vi "MCA_ConfigDialog.vi"(0 "测量最多花费的时间（秒）：":u16=3600, 1 "测量数据刷新频率（个/次）：":u32, 2 "数据文件路径":path, 3 "道数":enum32{"1024", "2048", "4096", "8192"}(radio), 4 "输入信号的极性：":enum32{"正", "负"}(radio), 5 "寻峰灵敏度：":u16=30 min=3 step=1, 6 "甄别前阈值":u16=200, 7 "甄别后阈值":u16=100) -> (14 "输入信号极性":bool, 16 "甄别后阈值 2":dbl=9000.0, 18 "甄别前阈值 2":dbl=10000.0, 20 "是否取消？":bool, 21 "道数最大值":i32, 23 "数据文件路径 2":path, 24 "寻峰灵敏度： 2":u32=30 min=3 step=1, 26 "测量数据刷新时间（个/次）： 2":u32, 27 "测量最多花费的时间（秒）： 2":u32=3600)   [LabVIEW 2014]
uses:
  <vilib>/Utility/config.llb/Write Key (U32).vi
  <vilib>/Utility/config.llb/Write Key (Path).vi
  <vilib>/Utility/config.llb/Write Key (I32).vi
  <vilib>/Utility/config.llb/Write Key (Boolean).vi
  <vilib>/Utility/config.llb/NI_LVConfig.lvlib
panel:
  in  "按钮_应用":bool
  in  "按钮_取消":bool
  in  "按钮_确定":bool
  in  "选项卡控件":enum32{"测量设置  ", "道数设置", "寻峰设置  ", "道宽修正  "}(tab)
  # "设置以下参数，使多道分析仪可以正常工作。多道分析仪只能同时测量单一极性的，\n幅度在一定范围内的核脉冲信号。"
  # "输入信号幅度的范围："
  # "（以8192道为标准）"
  # "（前阈值要大于后阈值）"
  # "多道分析仪可以改变道宽，以此来增加对信号幅度的分辨能力。\n道数越多，道宽相对越窄，对信号幅度的能力越高。"
  # "请设置多道分析仪总道数的大小："
  # "时间多道的寻峰功能，采用了利用二次多项式拟合各组数据点中的数据的办法进行\n寻峰。拟合中使用的数据点的数量由寻峰灵敏度指定。\n\n寻峰灵敏度过大，可能降低波峰的计数数值并改变其显示位置；灵敏度过小，可能会\n寻找出许多由噪声产生的毫无意义的杂峰。调整合适的灵敏度，使得多道可以识别出\n正确的峰位，并且使峰位的偏差和计数误差控制在最小的范围内。\n\n\n\n请设置时间多道的寻峰灵敏度："
  # "注：一般情况下，寻峰灵敏度要小于相应峰位的半高宽的一半。"
  # "请输入多道分析仪道宽修正数据的路径："
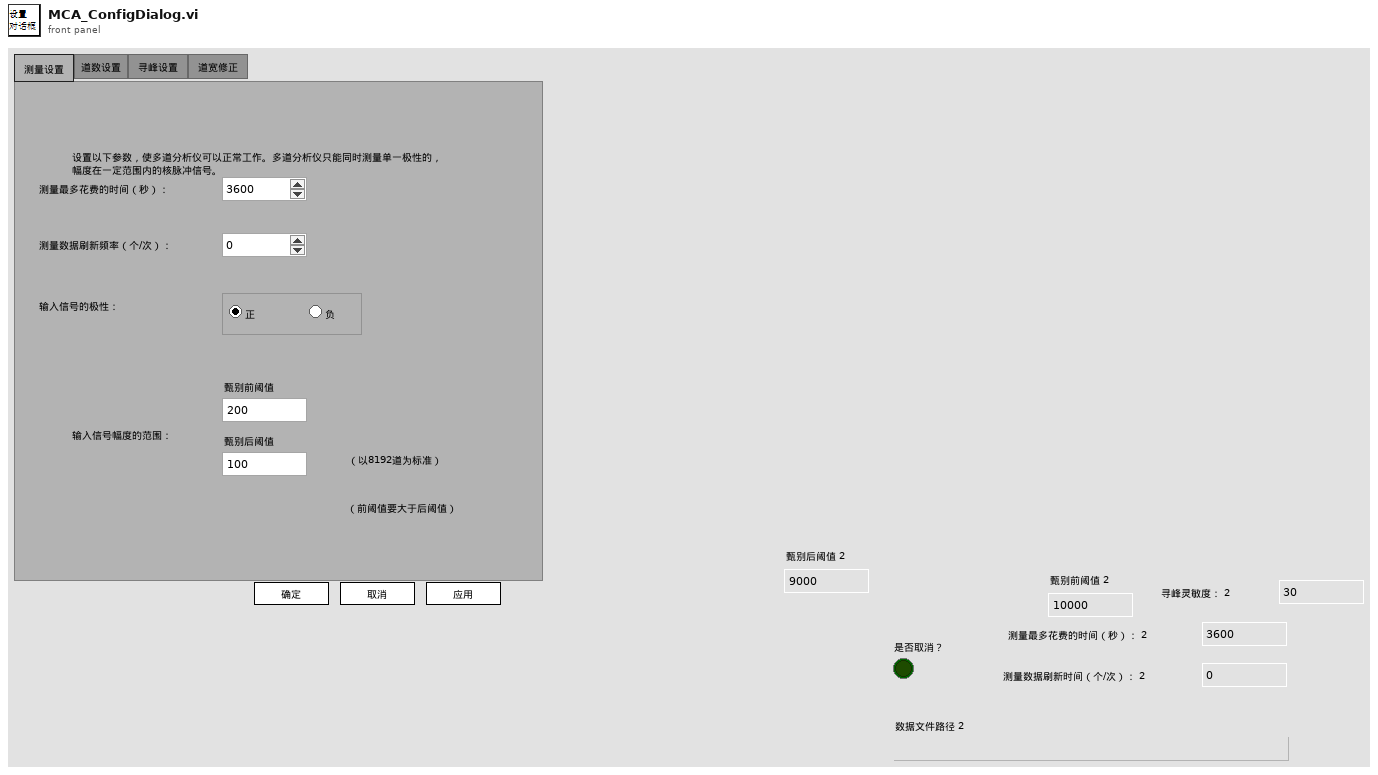
[diagram p1: front panel]
types:
  T1 = typedef "枚举常量_状态机.ctl" = enum16{"初始化", "等待", "完成"}
  T2 = enum8{"Enabled", "Disabled", "Disabled and Grayed Out"}
  T3 = typedef "NI_LVConfig.lvlib/Config Data RefNum.ctl" = refnum<k1>
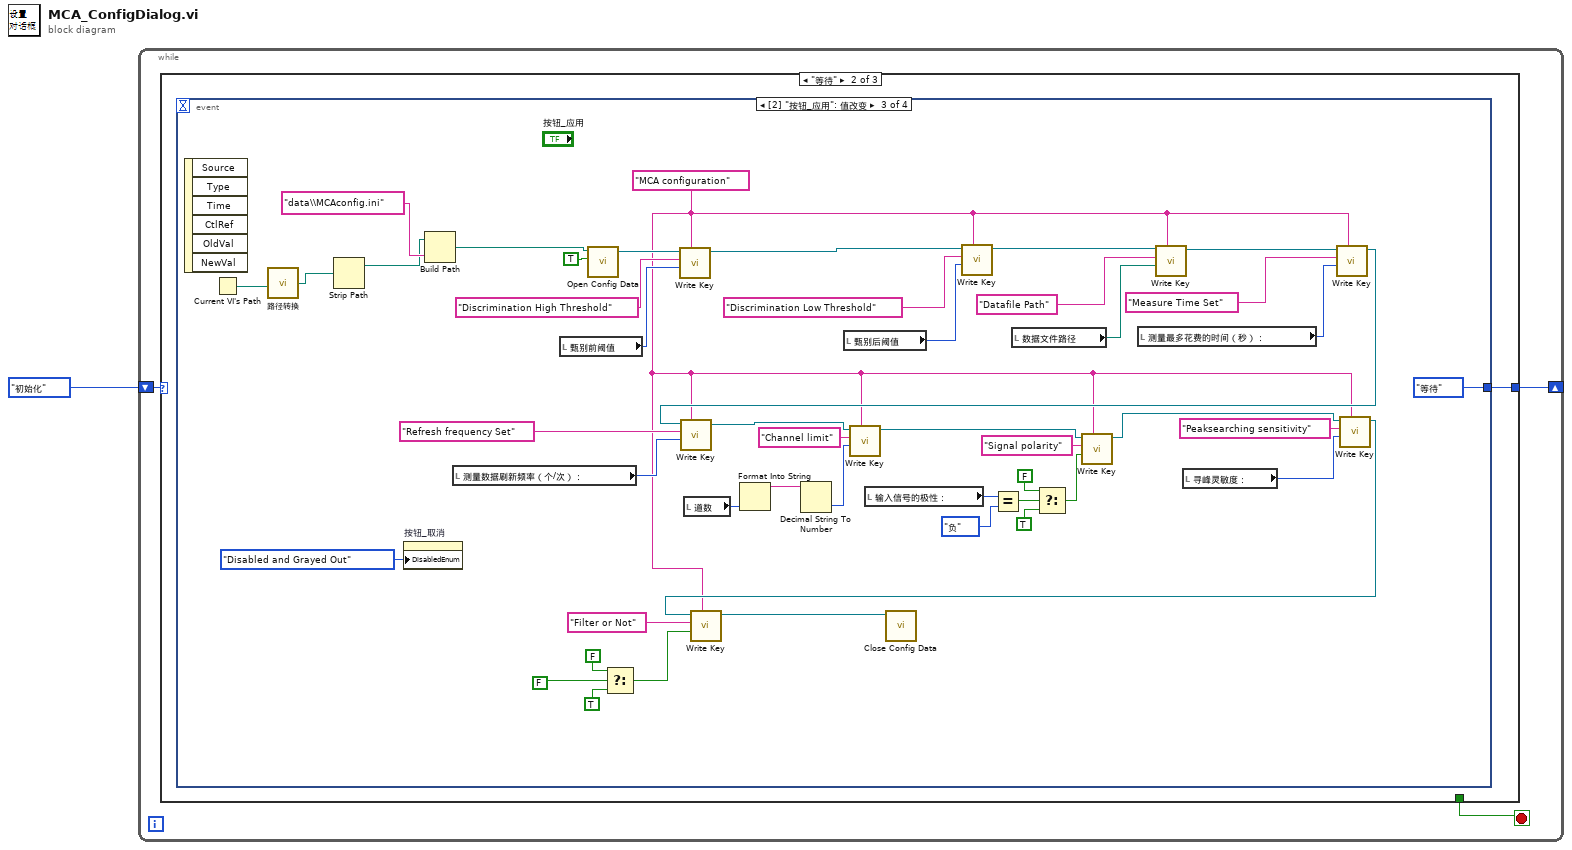
[diagram p0: block diagram]
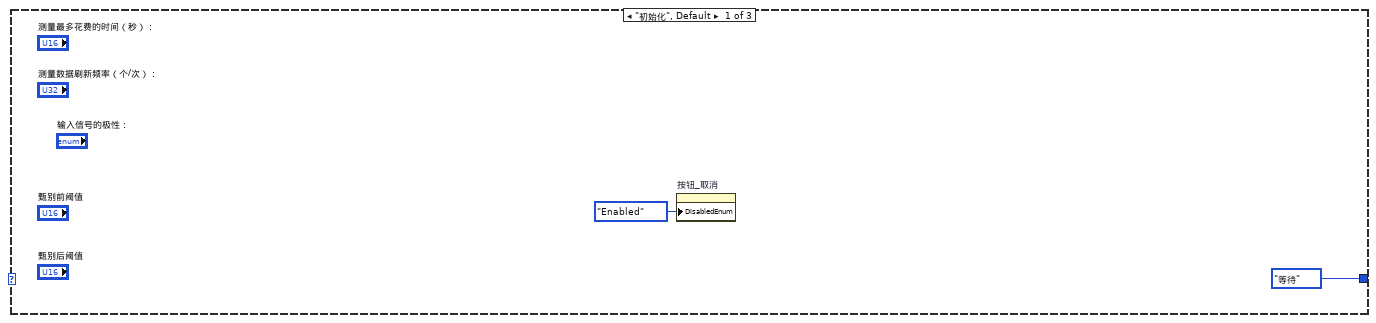
[diagram p2: hidden frame]
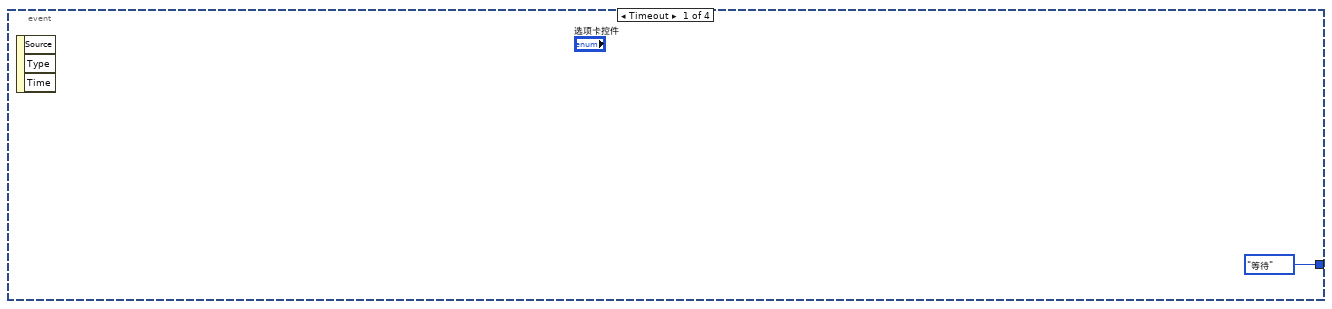
[diagram p3: hidden frame]
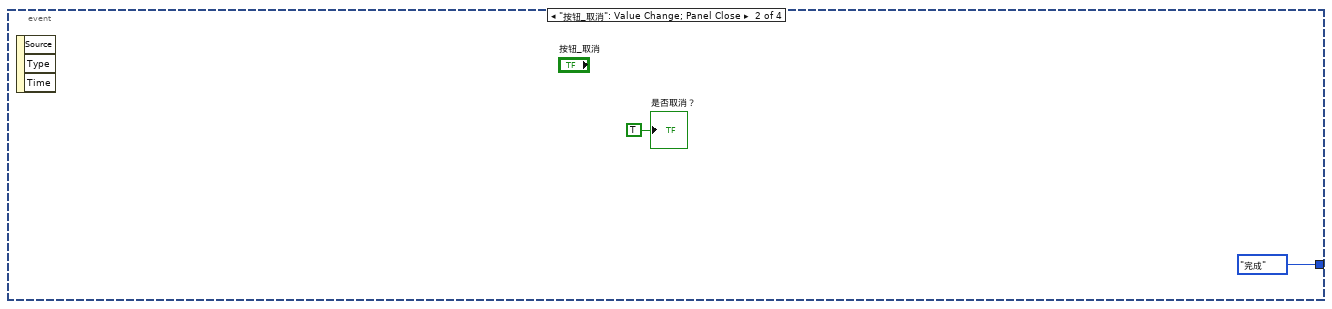
[diagram p4: hidden frame]
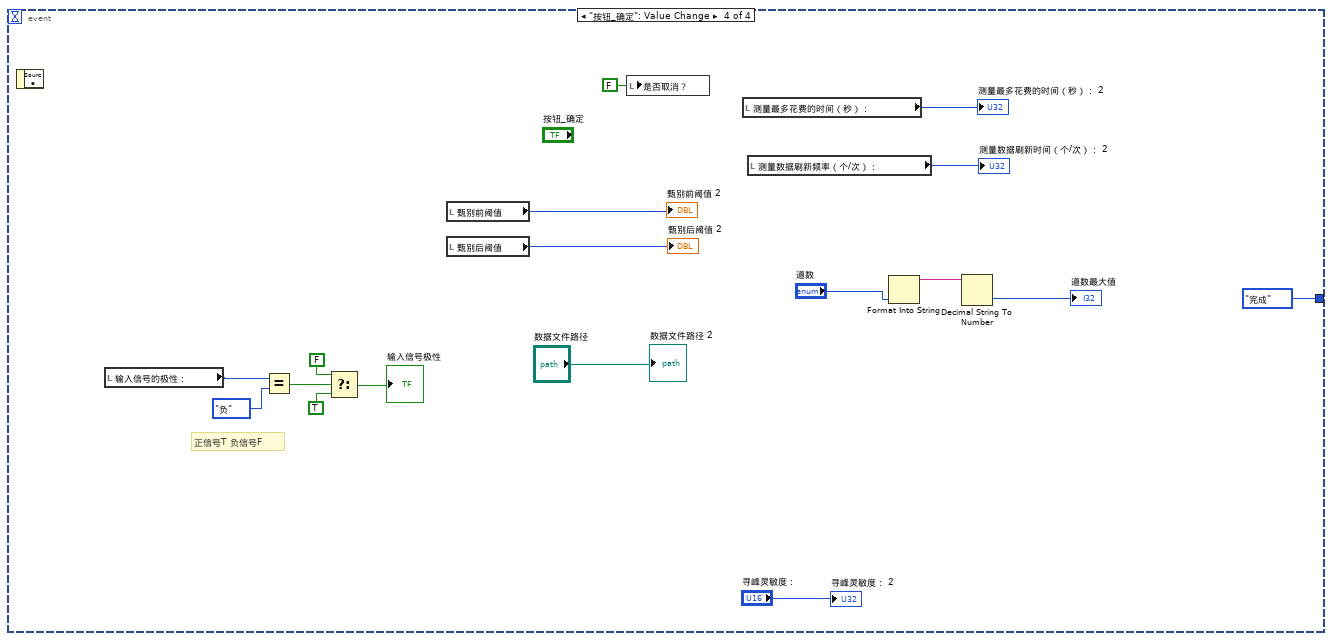
[diagram p5: hidden frame]
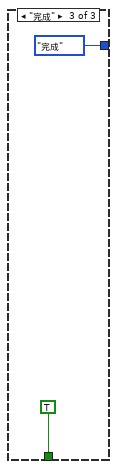
[diagram p6: hidden frame]
diagram:
  n1 = while {
    shift-right: [w2] -> _
    shift-left: 枚举常量_状态机."初始化" ("枚举") -> [w3]
    stop <- w4 stop-if-true
    n2 = case shown="\"等待\"" w3 {
      tunnel: [_ _ TRUE] -> w4
      tunnel: [枚举常量_状态机."等待" ("枚举") w7 枚举常量_状态机."完成" ("枚举")] -> w2
      frame "初始化", Default {
        n3 = property on="按钮_取消" class="Bool"("DisabledEnum"=T2."Enabled" ("禁用")) -> ()  [unwired: 2 in, 2 out]
      }
      frame "等待" {
        n4 = event shown="[2] \"按钮_应用\": 值改变" {
          selector: _ -> [_ _ _ _]
          dyn-events: _ -> [_ _ _ _]
          timeout: _ -> [_ _ _ _]
          tunnel: [枚举常量_状态机."等待" ("枚举") 枚举常量_状态机."完成" ("枚举") 枚举常量_状态机."等待" ("枚举") 枚举常量_状态机."完成" ("枚举")] -> w7
          event Timeout {
            n5 = event-data() -> ()  [unwired: 1 in, 3 out]
          }
          event "按钮_取消": Value Change; Panel Close {
            n6 = event-data() -> ()  [unwired: 1 in, 3 out]
            "是否取消？" <- TRUE ("是否取消？")
          }
          event "按钮_应用": Value Change {
            w20 = "MCA configuration" ("section")
            n7 = event-data() -> ()  [unwired: 1 in, 6 out]
            n8 = Current VI's Path() -> (path=w12:path)
            n9 = call "路径转换.vi"("input path"=w12) -> ("output path"=w11:path)
            n10 = Strip Path(path=w11) -> (stripped path=w13:path)  [unwired: 1 out]
            n11 = property on="按钮_取消" class="Bool"("DisabledEnum"=T2."Disabled and Grayed Out" ("禁用")) -> ()  [unwired: 2 in, 2 out]
            n12 = Build Path(base path=w13, name or relative path="data\\MCAconfig.ini" ("名称或相对路径")) -> (appended path=w23:path)
            n13 = local read "测量数据刷新频率（个/次）："() -> (w56:u32)
            n14 = local read "甄别前阈值"() -> (w52:u16)
            n15 = call <vilib>:"Open Config Data.vi"("create file if necessary (T)"=TRUE, "configuration file path"=w23) -> ("refnum"=w41:T3)  [unwired: 7 in, 2 out]
            n16 = Select(t=FALSE ("x = y?"), s=FALSE, f=TRUE) -> (s? t:f=w17:bool)
            n17 = call-poly <vilib>:"Write Key.vi"("section"=w20, "value"=w52, "key"="Discrimination High Threshold", "refnum"=w41) -> ("refnum out"=w43:T3)  [unwired: 5 in, 2 out]
            n18 = local read "道数"() -> (w33:enum32{"1024", "2048", "4096", "8192"})
            n19 = Format Into String(w33) -> (resulting string=w36:string)  [unwired: 3 in, 1 out]
            n20 = Decimal String To Number(string=w36) -> (number=w37:i32)  [unwired: 2 in, 1 out]
            n21 = local read "甄别后阈值"() -> (w53:u16)
            n22 = local read "输入信号的极性："() -> (w25:enum32{"正", "负"})
            n23 = call-poly <vilib>:"Write Key.vi"("section"=w20, "value"=w53, "key"="Discrimination Low Threshold", "refnum"=w43) -> ("refnum out"=w46:T3)  [unwired: 5 in, 2 out]
            n24 = Equal?(x=w25, y=enum32{"正", "负"}."负") -> (x = y?=w28:bool)
            n25 = local read "数据文件路径"() -> (w54:path)
            n26 = Select(t=FALSE ("x = y?"), s=w28, f=TRUE) -> (s? t:f=w24:bool)
            n27 = local read "测量最多花费的时间（秒）："() -> (w55:u16)
            n28 = call-poly <vilib>:"Write Key.vi"("section"=w20, "value"=w54, "key"="Datafile Path", "refnum"=w46) -> ("refnum out"=w47:T3)  [unwired: 5 in, 2 out]
            n29 = local read "寻峰灵敏度："() -> (w57:u16)
            n30 = call-poly <vilib>:"Write Key.vi"("section"=w20, "value"=w55, "key"="Measure Time Set", "refnum"=w47) -> ("refnum out"=w49:T3)  [unwired: 5 in, 2 out]
            n31 = call-poly <vilib>:"Write Key.vi"("section"=w20, "value"=w56, "key"="Refresh frequency Set", "refnum"=w49) -> ("refnum out"=w34:T3)  [unwired: 5 in, 2 out]
            n32 = call-poly <vilib>:"Write Key.vi"("section"=w20, "value"=w37, "key"="Channel limit", "refnum"=w34) -> ("refnum out"=w32:T3)  [unwired: 5 in, 2 out]
            n33 = call-poly <vilib>:"Write Key.vi"("section"=w20, "value"=w24, "key"="Signal polarity", "refnum"=w32) -> ("refnum out"=w30:T3)  [unwired: 5 in, 2 out]
            n34 = call-poly <vilib>:"Write Key.vi"("section"=w20, "value"=w57, "key"="Peaksearching sensitivity", "refnum"=w30) -> ("refnum out"=w21:T3)  [unwired: 5 in, 2 out]
            n35 = call-poly <vilib>:"Write Key.vi"("section"=w20, "value"=w17, "key"="Filter or Not", "refnum"=w21) -> ("refnum out"=w15:T3)  [unwired: 5 in, 2 out]
            n36 = call <vilib>:"Close Config Data.vi"("refnum"=w15) -> ()  [unwired: 9 in, 2 out]
          }
          event "按钮_确定": Value Change {
            # "正信号T 负信号F"
            n37 = event-data() -> ()  [unwired: 1 in, 1 out]
            n38 = local read "输入信号的极性："() -> (w59:enum32{"正", "负"})
            n39 = Equal?(x=w59, y=enum32{"正", "负"}."负") -> (x = y?=w62:bool)
            n40 = Select(t=FALSE ("x = y?"), s=w62, f=TRUE) -> (s? t:f=→"输入信号极性":bool)
            n41 = local read "甄别前阈值"() -> (→"甄别前阈值 2":u16)
            n42 = local read "甄别后阈值"() -> (→"甄别后阈值 2":u16)
            n43 = local write "是否取消？"(FALSE ("是否取消？")) -> ()
            n44 = local read "测量最多花费的时间（秒）："() -> (→"测量最多花费的时间（秒）： 2":u16)
            n45 = local read "测量数据刷新频率（个/次）："() -> (→"测量数据刷新时间（个/次）： 2":u32)
            n46 = Format Into String("道数") -> (resulting string=w70:string)  [unwired: 3 in, 1 out]
            n47 = Decimal String To Number(string=w70) -> (number=→"道数最大值":i32)  [unwired: 2 in, 1 out]
            "寻峰灵敏度： 2" <- "寻峰灵敏度："
            "数据文件路径 2" <- "数据文件路径"
          }
        }
      }
      frame "完成" {
      }
    }
  }
